vi "LinearQuadraticRegulator_GetU.vi"(11 "in LinearQuadraticRegulator":T2) -> (3 "U":T1)   [LabVIEW 2019, in "Trajectory_Library.lvlib"]
doc: "Returns the control input vector u.\n \nInputs:\n - LinearQuadraticRegulator -- controller data cluster\n\nOutputs:\n - U -- The control input."
uses:
  LINEAR_QUADRATIC_REGULATOR.ctl
  <vilib>/Analysis/Matrix/Datatypes/RealMatrix.ctl
  Trajectory_Library.lvlib
  <vilib>/Analysis/Matrix/NI_Matrix.lvlib
panel:
  # "Ref State <States,1>"
  # "Comp and capped \noutput <Inputs,1>"
  # "Controller gain\n<Inputs,States>"
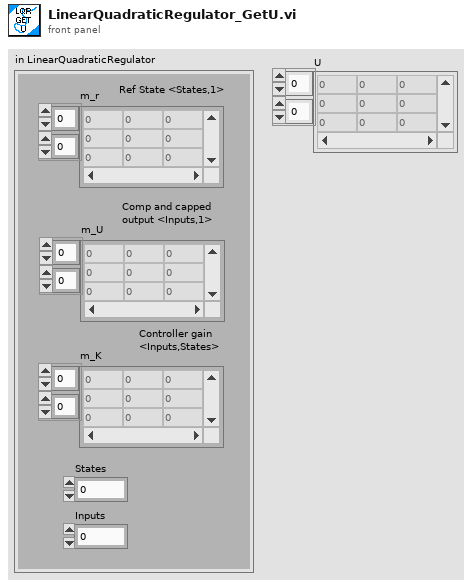
[diagram p1: front panel]
types:
  T1 = typedef "NI_Matrix.lvlib/RealMatrix.ctl" = dbl[][]
  T2 = typedef "Trajectory_Library.lvlib/LINEAR_QUADRATIC_REGULATOR.ctl" = cluster{"m_r":T1, "m_U":T1, "m_K":T1, "States":i32, "Inputs":i32}
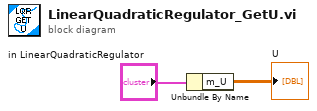
[diagram p0: block diagram]
diagram:
  n1 = Unbundle By Name("in LinearQuadraticRegulator") -> ("m_U"=→"U":T1)
